vi "DeferPanelUpdates.vi"(8 "error in (no error)":errorcluster, 10 "Defer Panel Updates":bool, 11 "VI Refnum In":refnum<vi>) -> (0 "error out":errorcluster, 3 "VI Refnum Out":refnum<vi>)   [LabVIEW 2020, in "Maui Manager.lvclass"]
uses:
  Maui Manager.lvclass
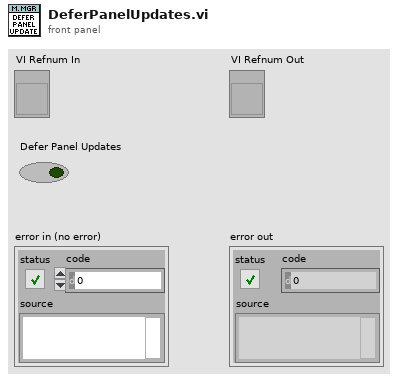
[diagram p1: front panel]
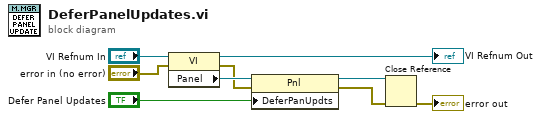
[diagram p0: block diagram]
diagram:
  n1 = property class="VI"(reference="VI Refnum In", error in="error in (no error)") -> (reference out=→"VI Refnum Out":refnum<vi>, error out=w3:errorcluster, "Panel"=w7:refnum<vi>)
  n2 = property class="Pnl"(reference=w7, error in=w3, "DeferPanUpdts"="Defer Panel Updates") -> (reference out=w5:refnum<vi>, error out=w2:errorcluster)
  n3 = Close Reference(reference=w5, error in (no error)=w2) -> (error out=→"error out":errorcluster)
